vi "FTW-Test-ActorAsk.vi"() -> (0 "Test Result":errorcluster)   [LabVIEW 2015]
uses:
  src/error/FTW-ERR-PrependExplanation.vi
  src/json/FTW-JSON-Object-SetElement-String.vi
  src/json/FTW-JSON-Object-GetElement-Bool.vi
  src/json/FTW-JSON-Object-GetElement-Integer.vi
  src/json/FTW-JSON-SerializeAndDestroy.vi
  src/actor/support/FTW-Actor-DynamicLaunchOptions.vi
  src/error/FTW-ERR-Ignore.vi
  src/error/FTW-ERR-ThrowError.vi
  src/actor/request/FTW-Request-InterpretResponse.vi
  lib/FTW-KernelFilepath.vi
  src/json/core/FTW-JSON-Core-EncodingFlags.vi
  src/reflection/FTW-Reflection-Type.vi
  codegen/xnode/json/fetch/FTW-JSON-Core-GetFlattenedValue.vi
  src/error/FTW-ERR-NoErrorConstant.vi
  src/socket/connector/FTW-Connector-Construct.vi
  src/time/FTW-Time-RelativeTimer.vi
  src/json/FTW-JSON-ObjectManip-AddPair.vi
  src/socket/connector/core/FTW-Connector-Core-Ask.vi
  codegen/xnode/FTW-Actor-Spawn.xnode
  src/core/type/FTW-Type-Actor-Connector.ctl
  codegen/xnode/FTW-JSON-Fetch.xnode
  codegen/xnode/FTW-Actor-Ask.xnode
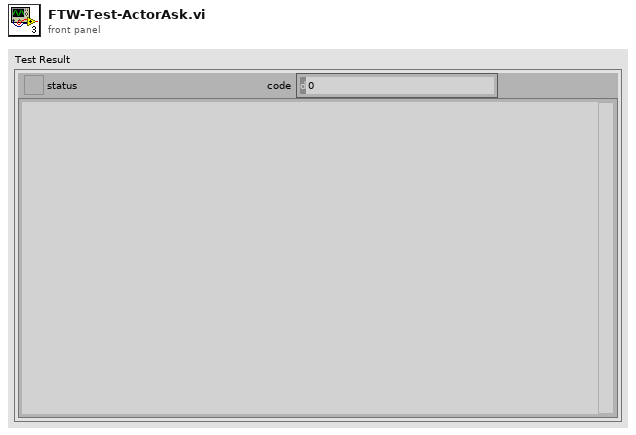
[diagram p1: front panel]
types:
  T1 = enum16{"Message is repeated verbatim", "Large message is repeated verbatim", "Fields are consumed", "Message is encoded"}[]
  T2 = typedef "FTW-Type-Actor-Connector.ctl" = refnum<data-value>
  T3 = cluster{"MessageField1":string, "MessageField2":string}
  T4 = cluster{"MessageFieldToKeep":string, "MessageFieldToConsume":string}
  T5 = typedef "FTW-Type-JSON.ctl" = refnum<data-value>
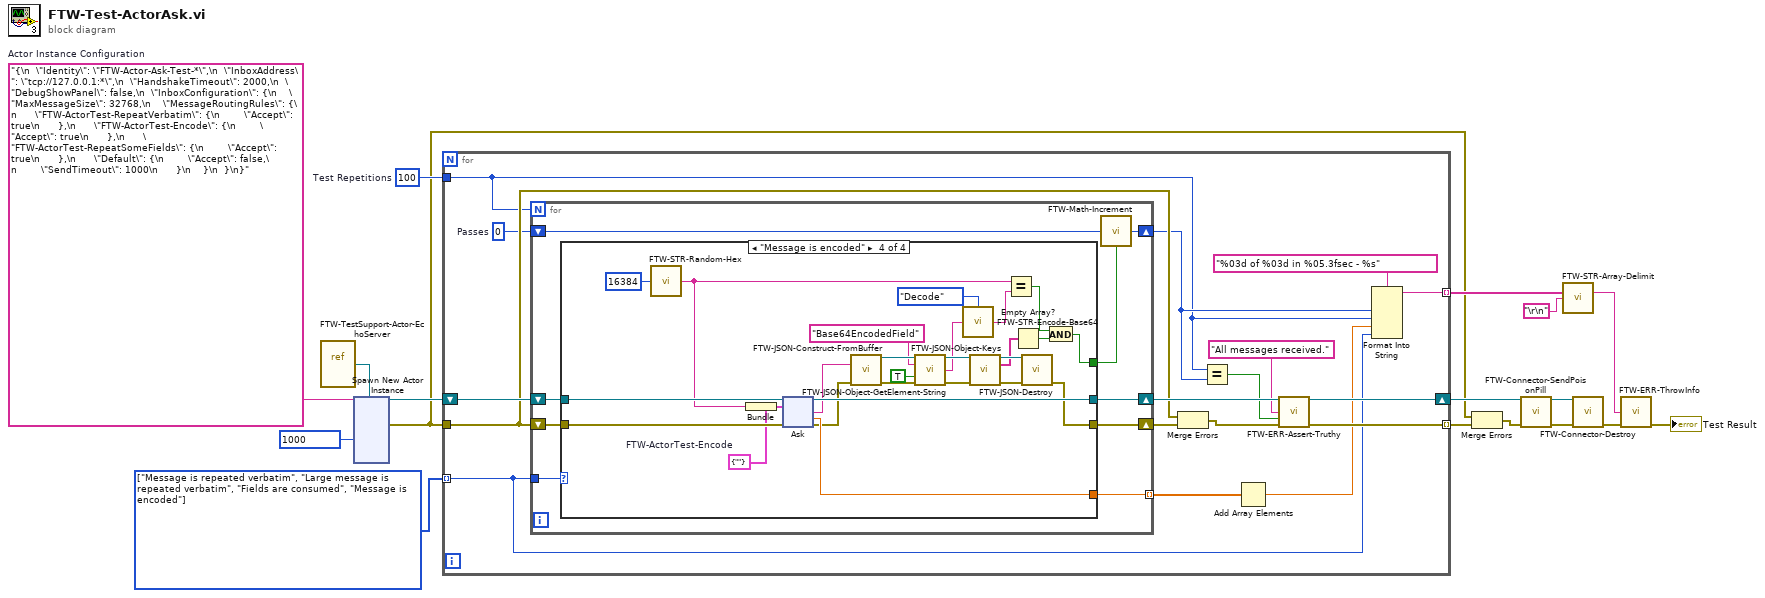
[diagram p0: block diagram]
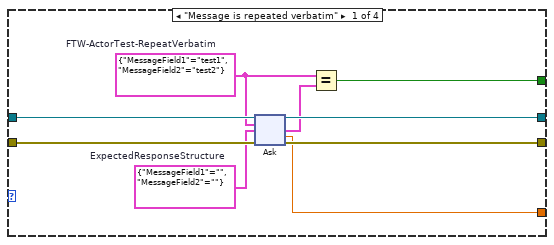
[diagram p2: hidden frame]
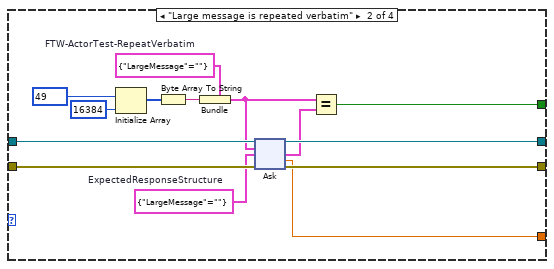
[diagram p3: hidden frame]
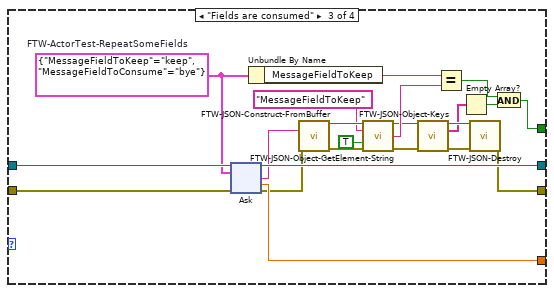
[diagram p4: hidden frame]
diagram:
  w4 = T1 [enum."Message is repeated verbatim", enum."Large message is repeated verbatim", enum."Fields are consumed", enum."Message is encoded"] items=["Message is repeated verbatim", "Large message is repeated verbatim", "Fields are consumed", "Message is encoded"]
  w6 = 100  # Test Repetitions
  w14 = "{\n  \"Identity\": \"FTW-Actor-Ask-Test-*\",\n  \"InboxAddress\": \"tcp://127.0.0.1:*\",\n  \"HandshakeTimeout\": 2000,\n  \"DebugShowPanel\": false,\n  \"InboxConfiguration\": {\n    \"MaxMessageSize\": 32768,\n    \"MessageRoutingRules\": {\n      \"FTW-ActorTest-RepeatVerbatim\": {\n        \"Accept\": true\n      },\n      \"FTW-ActorTest-Encode\": {\n        \"Accept\": true\n      },\n      \"FTW-ActorTest-RepeatSomeFields\": {\n        \"Accept\": true\n      },\n      \"Default\": {\n        \"Accept\": false,\n        \"SendTimeout\": 1000\n      }\n    }\n  }\n}"  # Actor Instance Configuration
  n1 = vi-ref "FTW-TestSupport-Actor-EchoServer.vi"() -> (w15:refnum<vi>)
  n2 = xnode "Spawn New Actor Instance"("Actor Instance Configuration"=w14, "Actor Instance Interface"=w15, "Idle Timeout"=1000) -> ("FTW Actor Connector"=w13:T2, "error out"=w3:errorcluster)  [unwired: 3 in, 2 out]
  n3 = for {
    shift-right: [w33] -> w16
    shift-left: w13 -> [w32]
    tunnel: [w20] -> w8 mode=indexing
    tunnel: w6 -> [w18]
    tunnel: w4 -> [w23] mode=indexing
    tunnel: w3 -> [w30]
    tunnel: [w25] -> w2 mode=indexing
    w28 = 0  # Passes
    n4 = for {
      N: w18 -> [_]
      tunnel: [w39] -> w31 mode=indexing
      shift-right: [w42] -> w33
      shift-left: w32 -> [w41]
      shift-right: [w37] -> w29
      shift-left: w30 -> [w40]
      tunnel: w23 -> [w38]
      shift-right: [w35] -> w24
      shift-left: w28 -> [w36]
      n5 = case shown="\"Message is encoded\"" w38 {
        tunnel: [w51 w140 w237 w280] -> w42
        tunnel: w41 -> [w50 w139 w236 w279]
        tunnel: w40 -> [w49 w138 w235 w278]
        tunnel: [w45 w134 w220 w266] -> w37
        tunnel: [w46 w135 w216 w262] -> w34
        tunnel: [w44 w133 w234 w277] -> w39
        frame "Message is repeated verbatim" {
          w48 = T3 {"MessageField1"="", "MessageField2"=""}  # ExpectedResponseStructure
          w43 = T3 {"MessageField1"="test1", "MessageField2"="test2"}  # FTW-ActorTest-RepeatVerbatim
          n6 = xnode "Ask"("FTW Actor Connector"=w50, "Request"=w43, "Response Type and Defaults"=w48, "error in"=w49) -> ("FTW Actor Connector out"=w51:T2, "Response"=w47:T3, "Roundtrip Time"=w44:dbl, "error out"=w45:errorcluster)  [unwired: 1 in]
          n7 = Equal?(x=w43, y=w47) -> (x = y?=w46:bool)
        }
        frame "Large message is repeated verbatim" {
          w137 = cluster{"LargeMessage":string} {"LargeMessage"=""}  # ExpectedResponseStructure
          w132 = cluster{"LargeMessage":string} {"LargeMessage"=""}  # FTW-ActorTest-RepeatVerbatim
          n8 = Initialize Array(u8 49, 16384 ("dimension size")) -> (w128:u8[])
          n9 = Byte Array To String(unsigned byte array=w128) -> (string=w127:string)
          n10 = Bundle(cluster=w132, "LargeMessage"=w127) -> (w131:cluster{"LargeMessage":string})
          n11 = xnode "Ask"("FTW Actor Connector"=w139, "Request"=w131, "Response Type and Defaults"=w137, "error in"=w138) -> ("FTW Actor Connector out"=w140:T2, "Response"=w136:cluster{"LargeMessage":string}, "Roundtrip Time"=w133:dbl, "error out"=w134:errorcluster)  [unwired: 1 in]
          n12 = Equal?(x=w131, y=w136) -> (x = y?=w135:bool)
        }
        frame "Fields are consumed" {
          w233 = T4 {"MessageFieldToKeep"="keep", "MessageFieldToConsume"="bye"}  # FTW-ActorTest-RepeatSomeFields
          n13 = xnode "Ask"("FTW Actor Connector"=w236, "Request"=w233, "error in"=w235) -> ("FTW Actor Connector out"=w237:T2, "Response"=w231:string, "Roundtrip Time"=w234:dbl, "error out"=w221:errorcluster)  [unwired: 2 in]
          n14 = Unbundle By Name(w233) -> ("MessageFieldToKeep"=w232:string)
          n15 = call "FTW-JSON-Construct-FromBuffer.vi"("JSON String (UTF-8)"=w231, "error in"=w221) -> ("JSON"=w230:T5, "error out"=w229:errorcluster)  [unwired: 12 in]
          n16 = call "FTW-JSON-Object-GetElement-String.vi"("JSON"=w230, "Key"="MessageFieldToKeep", "Consume Value"=TRUE, "error in"=w229) -> ("JSON out"=w225:T5, "Value"=w227:string, "error out"=w224:errorcluster)  [unwired: 8 in, 1 out]
          n17 = call "FTW-JSON-Object-Keys.vi"("JSON"=w225, "error in"=w224) -> ("JSON out"=w223:T5, "Keys"=w219:string[], "error out"=w222:errorcluster)  [unwired: 11 in]
          n18 = Equal?(x=w232, y=w227) -> (x = y?=w217:bool)
          n19 = Empty Array?(array=w219) -> (empty?=w218:bool)
          n20 = call "FTW-JSON-Destroy.vi"("JSON"=w223, "error in"=w222) -> ("error out"=w220:errorcluster)  [unwired: 13 in]
          n21 = And(x=w217, y=w218) -> (x .and. y?=w216:bool)
        }
        frame "Message is encoded" {
          w259 = cluster{"MessageFieldToEncode":string} {"MessageFieldToEncode"=""}  # FTW-ActorTest-Encode
          n22 = call "FTW-STR-Random-Hex.vi"("String Length"=16384) -> ("Random Hex String"=w258:string)  [unwired: 3 in]
          n23 = Bundle(cluster=w259, "MessageFieldToEncode"=w258) -> (w260:cluster{"MessageFieldToEncode":string})
          n24 = xnode "Ask"("FTW Actor Connector"=w279, "Request"=w260, "error in"=w278) -> ("FTW Actor Connector out"=w280:T2, "Response"=w276:string, "Roundtrip Time"=w277:dbl, "error out"=w267:errorcluster)  [unwired: 2 in]
          n25 = call "FTW-JSON-Construct-FromBuffer.vi"("JSON String (UTF-8)"=w276, "error in"=w267) -> ("JSON"=w275:T5, "error out"=w274:errorcluster)  [unwired: 12 in]
          n26 = call "FTW-JSON-Object-GetElement-String.vi"("JSON"=w275, "Key"="Base64EncodedField", "Consume Value"=TRUE, "error in"=w274) -> ("JSON out"=w271:T5, "Value"=w256:string, "error out"=w270:errorcluster)  [unwired: 8 in, 1 out]
          n27 = call "FTW-STR-Encode-Base64.vi"("Input"=w256, "Direction"=enum16{"Encode", "Decode"}."Decode") -> ("Output"=w255:string)
          n28 = call "FTW-JSON-Object-Keys.vi"("JSON"=w271, "error in"=w270) -> ("JSON out"=w269:T5, "Keys"=w265:string[], "error out"=w268:errorcluster)  [unwired: 11 in]
          n29 = Equal?(x=w258, y=w255) -> (x = y?=w263:bool)
          n30 = Empty Array?(array=w265) -> (empty?=w264:bool)
          n31 = call "FTW-JSON-Destroy.vi"("JSON"=w269, "error in"=w268) -> ("error out"=w266:errorcluster)  [unwired: 13 in]
          n32 = And(x=w263, y=w264) -> (x .and. y?=w262:bool)
        }
      }
      n33 = call "FTW-Math-Increment.vi"("Initial Value"=w36, "Increment?"=w34) -> ("Final Value"=w35:i32)
    }
    n34 = Merge Errors(w30, w29) -> (w26:errorcluster)
    n35 = Equal?(x=w18, y=w24) -> (x = y?=w27:bool)
    n36 = Add Array Elements(numeric array=w31) -> (sum=w22:dbl)
    n37 = call "FTW-ERR-Assert-Truthy.vi"("Assertion"="All messages received.", "Assertion holds true?"=w27, "error in"=w26) -> ("error out"=w25:errorcluster)  [unwired: 12 in]
    n38 = Format Into String(format string="%03d of %03d in %05.3fsec - %s", w24, w18, w22, w23) -> (resulting string=w20:string)  [unwired: 2 in, 1 out]
  }
  n39 = Merge Errors(w3, w2) -> (w1:errorcluster)
  n40 = call "FTW-Connector-SendPoisonPill.vi"("Actor Connector"=w16, "error in"=w1) -> ("Actor Connector out"=w17:T2, "error out"=w5:errorcluster)  [unwired: 10 in, 2 out]
  n41 = call "FTW-STR-Array-Delimit.vi"("Array of Strings"=w8, "Delimiter"="\r\n") -> ("Delimited String"=w7:string)  [unwired: 13 in]
  n42 = call "FTW-Connector-Destroy.vi"("Actor Connector"=w17, "error in"=w5) -> ("error out"=w11:errorcluster)  [unwired: 13 in]
  n43 = call "FTW-ERR-ThrowInfo.vi"("Informational Message"=w7, "error in"=w11) -> ("error out"=→"Test Result":errorcluster)  [unwired: 13 in]
